vi "V50 Report Results (SubVI).vi"(0 "NI_report in":refnum<class "NI_report.lvclass">, 5 "SampleID":string, 11 "error in (no error)":errorcluster) -> (4 "NI_report out":refnum<class "NI_report.lvclass">, 15 "error out":errorcluster)   [LabVIEW 2015]
uses:
  <vilib>/Utility/NIReport.llb/NI_report.lvclass
panel:
  out "recordset data":string[][](array[string])
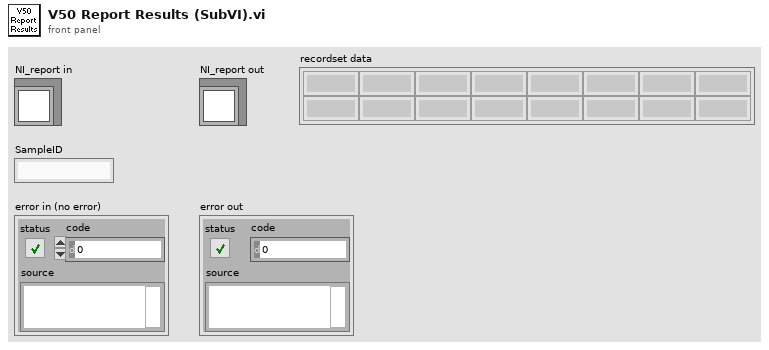
[diagram p1: front panel]
types:
  T1 = cluster{"position (excel)":cluster{"row":i32, "column":i32}, "name (excel)":string, "bookmark (word)":string}
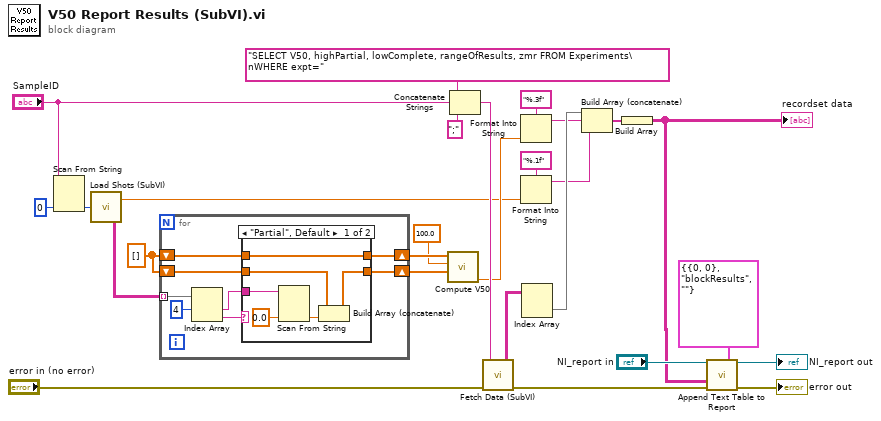
[diagram p0: block diagram]
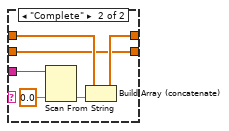
[diagram p2: hidden frame]
diagram:
  w5 = sgl[] []
  n1 = Scan From String(input string="SampleID", default 1=0 ("Record #")) -> (output 1=w16:i32)  [unwired: 3 in, 3 out]
  n2 = call "Load Shots (SubVI).vi"("Record #"=w16) -> ("Shot Array"=w8:string[][], "AvgDef"=w3:dbl)  [unwired: 2 in]
  n3 = for {
    tunnel: w8 -> [w35] mode=indexing
    shift-right: [w31] -> w7
    shift-left: w5 -> [w28]
    shift-right: [w30] -> w6
    shift-left: w5 -> [w29]
    n4 = Index Array(array=w35, index #1=4 ("index")) -> (element #1=w32:string, element #2=w33:string)  [unwired: 1 in]
    n5 = case shown="\"Partial\", Default" w33 {
      tunnel: w32 -> [w41 w47]
      tunnel: [w39 w42] -> w31
      tunnel: [w36 w44] -> w30
      tunnel: w29 -> [w36 w43]
      tunnel: w28 -> [w37 w42]
      frame "Partial", Default {
        n6 = Scan From String(input string=w41, default 1=sgl 0.0 ("default value 1")) -> (output 1=w40:sgl)  [unwired: 3 in, 3 out]
        n7 = Build Array (concatenate)(w37, w40) -> (w39:sgl[])
      }
      frame "Complete" {
        n8 = Scan From String(input string=w47, default 1=sgl 0.0 ("default value 1")) -> (output 1=w46:sgl)  [unwired: 3 in, 3 out]
        n9 = Build Array (concatenate)(w43, w46) -> (w44:sgl[])
      }
    }
  }
  n10 = call "Compute V50.vi"("Partial"=w7, "Maximum Deviation"=sgl 100.0, "Complete"=w6) -> ("velSTDEV"=w9:sgl)  [unwired: 4 out]
  n11 = Concatenate Strings("SELECT V50, highPartial, lowComplete, rangeOfResults, zmr FROM Experiments\nWHERE expt=" ("query string"), "SampleID", ";" ("string")) -> (w25:string)
  n12 = call "Fetch Data (SubVI).vi"("error IN"="error in (no error)", "query string"=w25) -> ("error OUT"=w19:errorcluster, "recordset data"=w14:string[][])  [unwired: 4 out]
  n13 = Format Into String(format string="%.3f", w9) -> (resulting string=w12:string)  [unwired: 2 in, 1 out]
  n14 = Format Into String(format string="%.1f", w3) -> (resulting string=w2:string)  [unwired: 2 in, 1 out]
  n15 = Index Array(array=w14) -> (element=w13:string[])  [unwired: 2 in]
  n16 = Build Array (concatenate)(w13, w12, w2) -> (w15:string[])
  n17 = Build Array(w15) -> (w11:string[][])
  "recordset data" <- w11
  n18 = call-dynamic "Append Text Table to Report.vi"("report in"="NI_report in", "MS Office parameters"=T1 {"position (excel)"={"row"=0, "column"=0}, "name (excel)"="blockResults", "bookmark (word)"=""}, "text data"=w11, "error in (no error)"=w19) -> ("report out"=→"NI_report out":refnum<class "NI_report.lvclass">, "error out"=→"error out":errorcluster)  [unwired: 8 in, 2 out]
